vi "Init.vi"(8 "error in (no error)":errorcluster) -> (0 "error out":errorcluster, 3 "Stand out":refnum<class "Stand.lvclass">)   [LabVIEW 2019, in "Stand.lvclass"]
uses:
  Stand.lvclass
  Database_Postgress_class/Database_Postgress.lvclass
  C:/Users/ANENKOV_V1/Desktop/src/DatabaseInterface_class/DatabaseInterface.lvclass
  Logger_class/Logger.lvclass
  ConfigJSON_class/ConfigJSON.lvclass
  C:/Users/ANENKOV_V1/Desktop/src/ConfigInterface_class/ConfigInterface.lvclass
  Proccess_class/TAGs.ctl
  Database_Postgress_class/Connection Info.ctl
  ConfigJSON_class/ConfigJSON.lvclass/ConfigJSON.ctl
  FPGA API Concrete_class/FPGA API Concrete.lvclass
  C:/Users/ANENKOV_V1/Desktop/src/FPGA_API_class/FPGA API.lvclass
  DatabaseInterface_class/DatabaseInterface.lvclass
  Modbus_class/ModbusSp.lvclass
  SV_Puplisher_class/SV_Publisher.lvclass
  Proccess_class/Proccess.lvclass
  FPGA API Mock_class/FPGA API Mock.lvclass
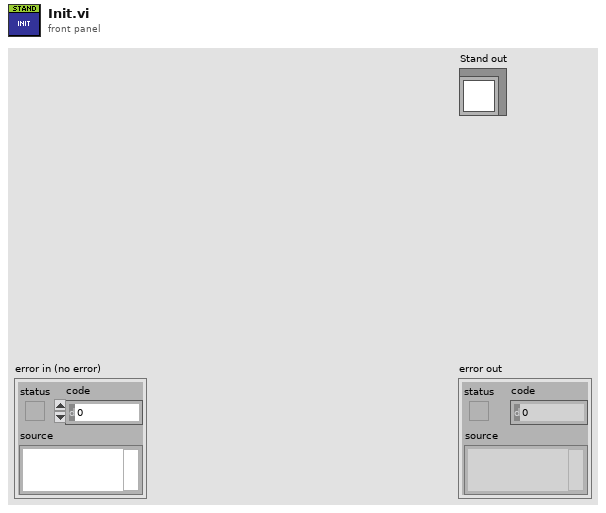
[diagram p1: front panel]
types:
  T1 = typedef "DatabaseInterface.lvclass/Connection Info.ctl" = cluster{"IP_Address":string, "Port":u16, "Timeout":i32, "User":string, "Password":string, "Database":string}
  T2 = typedef "Proccess.lvclass/TAGs.ctl" = cluster{"TAG":string, "PTAG":string, "DESC":string}
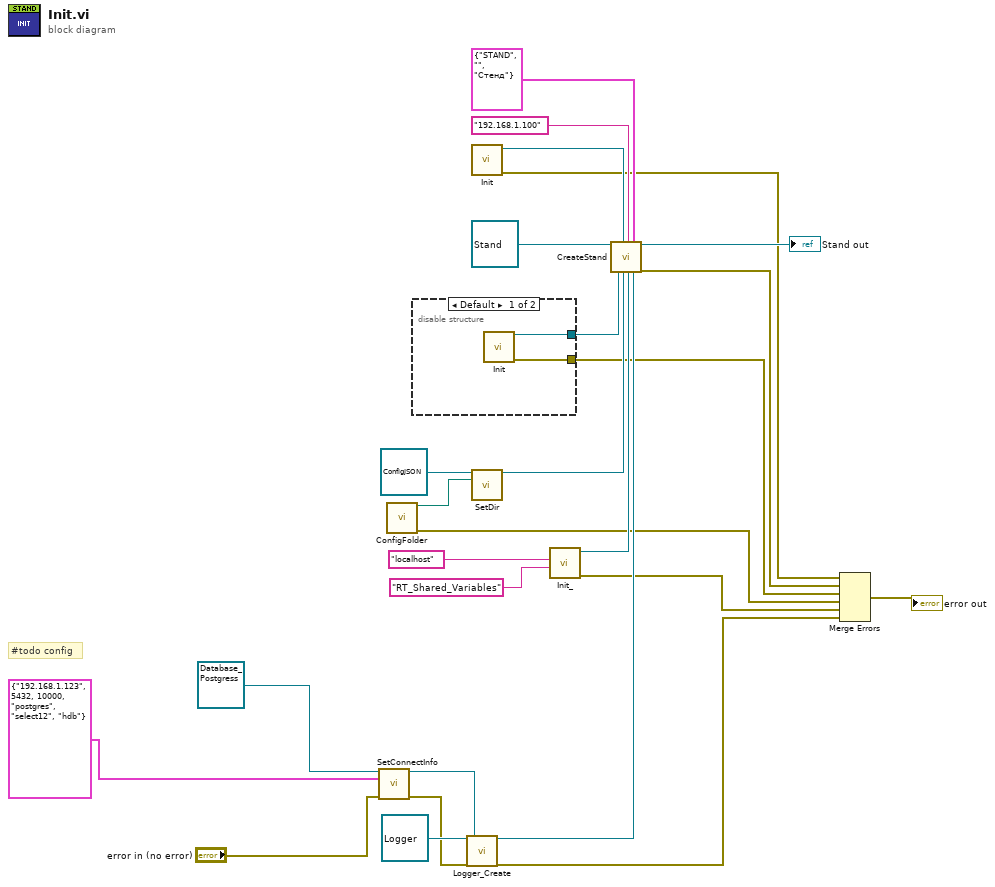
[diagram p0: block diagram]
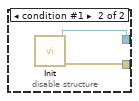
[diagram p2: hidden frame]
diagram:
  # "#todo config"
  n1 = call-dynamic "SetConnectInfo.vi"("reference in"=refnum<class "Database_Postgress.lvclass"> refnum, "Connection Info"=T1 {"IP_Address"="192.168.1.123", "Port"=5432, "Timeout"=10000, "User"="postgres", "Password"="select12", "Database"="hdb"}, "error in (no error)"="error in (no error)") -> ("reference out"=w23:refnum<class "Database_Postgress.lvclass">, "error out"=w22:errorcluster)  [unwired: 11 in]
  n2 = call "ConfigFolder.vi"() -> ("dup path"=w20:path, "error out"=w7:errorcluster)  [unwired: 14 in]
  n3 = disable-structure shown="Default" {
    disable-tunnel: [w28 w29] -> w3
    disable-tunnel: [w27 w30] -> w2
    frame condition #0 (active) {
      n4 = call "Init.vi"() -> ("FPGA API out"=w28:refnum<class "FPGA API Concrete.lvclass">, "error out"=w27:errorcluster)  [unwired: 14 in]
    }
    frame condition #1 {
      n5 = call "Init.vi"() -> ("FPGA API out"=w29:refnum<class "FPGA API Mock.lvclass">, "error out"=w30:errorcluster)  [unwired: 14 in]
    }
  }
  n6 = call "Logger_Create.vi"("reference in"=refnum<class "Logger.lvclass"> refnum, "error in (no error)"=w22, "DatabaseInterface"=w23) -> ("reference out"=w11:refnum<class "Logger.lvclass">, "error out"=w5:errorcluster)  [unwired: 15 in]
  n7 = call "Init.vi"() -> ("error out"=w9:errorcluster, "ModbusSp out"=w14:refnum<class "ModbusSp.lvclass">)  [unwired: 10 in]
  n8 = call "SetDir.vi"("reference in"=refnum<class "ConfigJSON.lvclass"> refnum ("ConfigJSON"), "Config Dir"=w20) -> ("JSON"=w13:refnum<class "ConfigJSON.lvclass">)  [unwired: 13 in]
  n9 = call "Init_.vi"("lib"="RT_Shared_Variables", "host"="localhost") -> ("error out"=w6:errorcluster, "SV_Publisher out"=w12:refnum<class "SV_Publisher.lvclass">)  [unwired: 8 in]
  n10 = call "CreateStand.vi"("Stand in"=refnum<class "Stand.lvclass"> refnum, "FPGA API"=w3, "Modbus"=w14, "ConfigInterface"=w13, "NV Addres"="192.168.1.100", "SV_Publisher"=w12, "Tags"=T2 {"TAG"="STAND", "PTAG"="", "DESC"="Стенд"}, "Logger"=w11) -> ("Stand out"=→"Stand out":refnum<class "Stand.lvclass">, "error out"=w8:errorcluster)  [unwired: 10 in]
  n11 = Merge Errors(w9, w8, w2, w7, w6, w5) -> (→"error out":errorcluster)
